vi "open handle.vi"(8 "error in (no error)":errorcluster caption="错误输入（无错误）", 11 "http client 输入":refnum<class "http client.lvclass">) -> (0 "error out":errorcluster caption="错误输出", 3 "http client 输出":refnum<class "http client.lvclass">)   [LabVIEW 2016, in "数据传输系统-06.lvlib" / "update.lvlib" / "http client.lvclass"]
uses:
  http client.lvclass
  http client.lvclass/http client.ctl
  <vilib>/httpClient/LabVIEWHTTPClient.lvlib
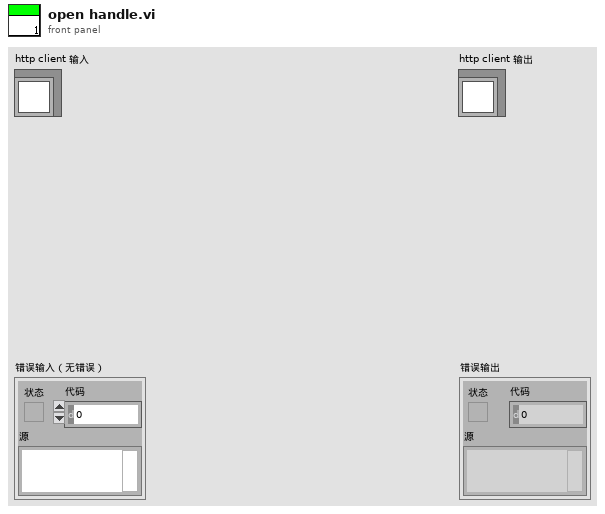
[diagram p1: front panel]
types:
  T1 = typedef "LabVIEWHTTPClient.lvlib/ClientHandle.ctl" = refnum<k1>
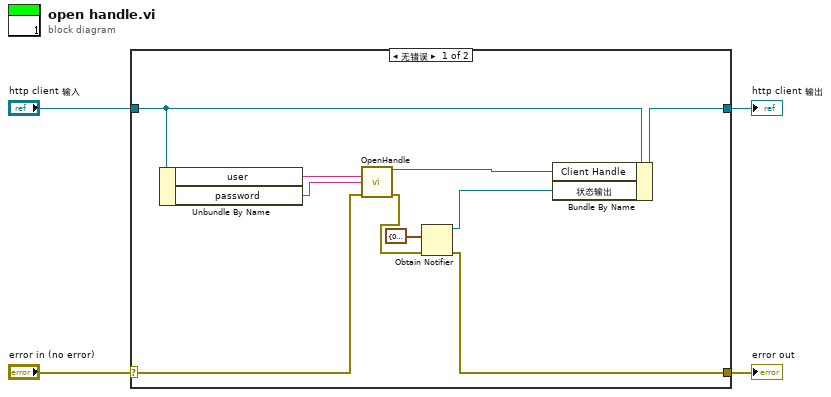
[diagram p0: block diagram]
diagram:
  n1 = case shown="无错误" "error in (no error)" {
    selector: "error in (no error)" -> [w11 w16]
    tunnel: [w6 w16] -> w3
    tunnel: [w10 w15] -> w1
    tunnel: "http client 输入" -> [w14 w15]
    frame No Error {
      n2 = Unbundle By Name(w14) -> ("user"=w13:string, "password"=w12:string)
      n3 = call <vilib>:"OpenHandle.vi"("username"=w13, "password"=w12, "error in (no error)"=w11) -> ("client handle out"=w9:T1, "error out"=w7:errorcluster)  [unwired: 11 in]
      n4 = Obtain Notifier(notification data type=cluster{"文件大小":i64, "已下载大小":i64, "滑动杆":dbl} {"文件大小"=0, "已下载大小"=0, "滑动杆"=0.0}, error in (no error)=w7) -> (notifier out=w5:refnum<notifier>, error out=w6:errorcluster)  [unwired: 2 in, 1 out]
      n5 = Bundle By Name(cluster=w14, "Client Handle"=w9, "状态输出"=w5) -> (w10:refnum<class "http client.lvclass">)
    }
    frame Error {
    }
  }
  "error out" <- w3
  "http client 输出" <- w1
